vi "FGV_Undo Redo.vi"(7 "Action":T1, 8 "error in":errorcluster, 10 "State In":string, 11 "menu reference":refnum<k9>) -> (0 "error out":errorcluster, 1 "Have Changes":bool, 2 "State Out":string)   [LabVIEW 2020, in "lv_icon.lvlib" / "History.lvclass"]
doc: "Circular buffer used to maintain states of the icon for the purpose of being able to perform Undo and Redo.\n\nAfter initialization, it is expected the first \"Add\" will establish the initial condition."
uses:
  History.lvclass
  History.lvclass/History.ctl
  Undo Redo Action.ctl
panel:
  out "Had Roll Over":bool
  out "Available Redo":i32
  out "Available Undo":i32
  out "Current Pointer":i32
  out "Buffer":string[](array[string])
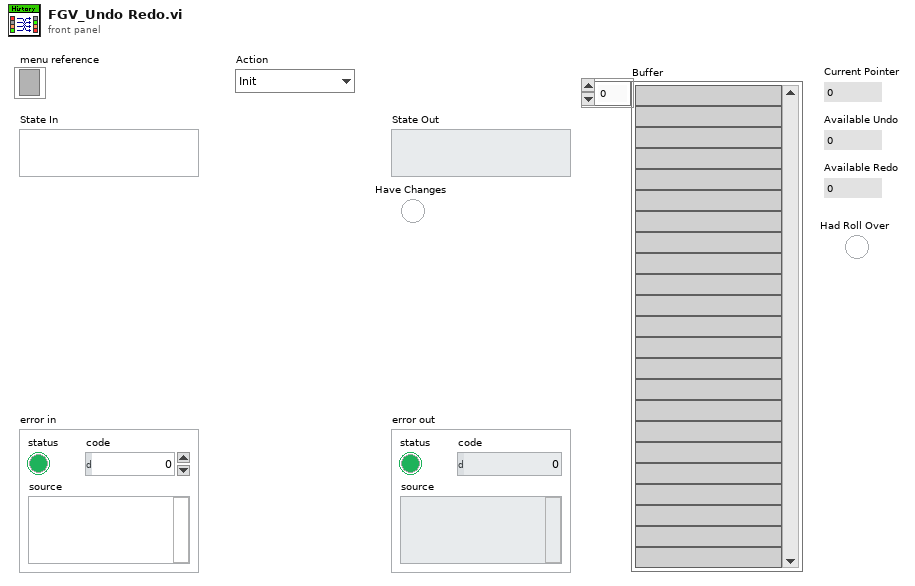
[diagram p1: front panel]
types:
  T1 = typedef "lv_icon.lvlib/History.lvclass/Undo Redo Action.ctl" = enum16{"Init", "Add", "Undo", "Redo", "Current State"}
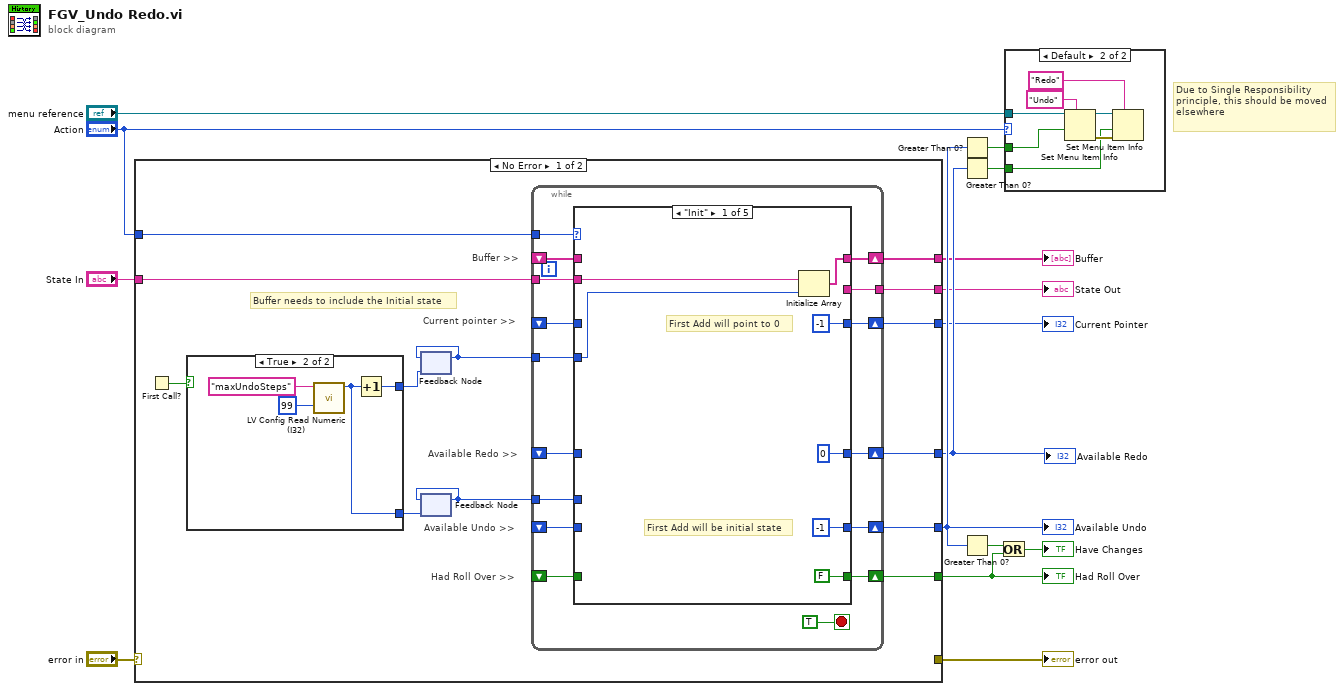
[diagram p0: block diagram]
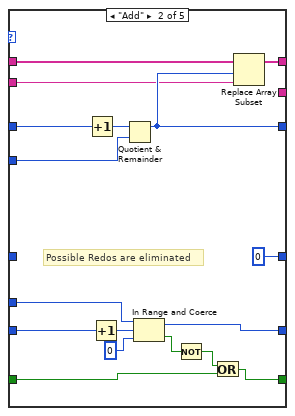
[diagram p3: hidden frame]
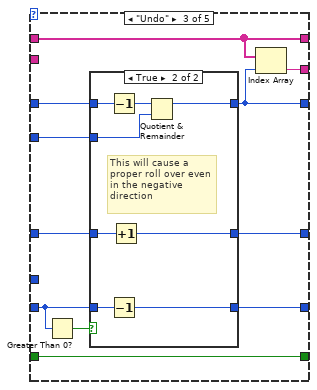
[diagram p4: hidden frame]
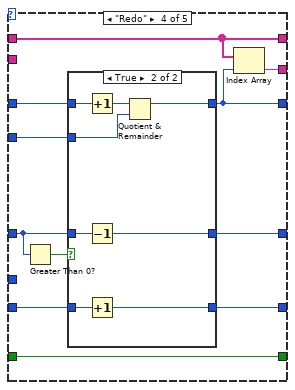
[diagram p6: hidden frame]
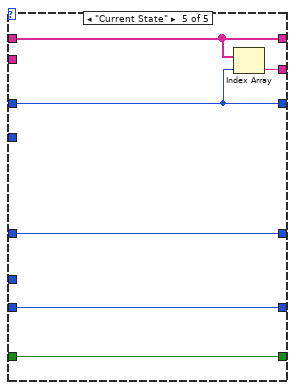
[diagram p8: hidden frame]
diagram:
  # "Due to Single Responsibility principle, this should be moved elsewhere"
  n1 = case shown="No Error" "error in" {
    selector: "error in" -> [_ w123]
    tunnel: [_ w123] -> w13
    tunnel: "Action" -> [w28 _]
    tunnel: "State In" -> [w27 _]
    tunnel: [w26 _] -> w3
    tunnel: [w23 _] -> w12
    tunnel: [w22 _] -> w1
    tunnel: [w20 _] -> w15
    tunnel: [w19 _] -> w2
    tunnel: [w16 _] -> w5
    frame No Error {
      # "Had Roll Over >>"
      # "Buffer needs to include the Initial state"
      # "Buffer >>"
      # "Available Undo >>"
      # "Available Redo >>"
      # "Current pointer >>"
      n2 = First Call?() -> (First Call?: T/F=w25:bool)
      n3 = case shown="True" w25 {
        tunnel: [_ w120] -> w21
        tunnel: [_ w119] -> w18
        frame False {
        }
        frame True {
          n4 = call <resource>:"LV Config Read Numeric (I32).vi"("default value"=99, "key"="maxUndoSteps") -> ("value"=w119:i32)  [unwired: 3 in, 2 out]
          n5 = Increment(x=w119) -> (x+1=w120:i32)
        }
      }
      n6 = feedback #1(w21) -> (w24:i32)
      n7 = feedback-in #1(w24) -> ()
      n8 = feedback #2(w18) -> (w17:i32)
      n9 = feedback-in #2(w17) -> ()
      n10 = while {
        tunnel: w28 -> [w43]
        shift-right: [w42] -> w19
        shift-left: _ -> [w41]
        tunnel: w27 -> [w40]
        shift-right: [w39] -> w22
        shift-left: _ -> [w38]
        shift-right: [w36] -> w23
        shift-left: _ -> [w37]
        tunnel: [w35] -> w26
        tunnel: w24 -> [w34]
        shift-right: [w32] -> w20
        shift-left: _ -> [w33]
        tunnel: w17 -> [w31]
        shift-right: [w29] -> w16
        shift-left: _ -> [w30]
        stop <- TRUE stop-if-true
        n11 = case shown="\"Init\"" w43 {
          tunnel: [w50 w68 w70 w100 w117] -> w42
          tunnel: w41 -> [_ w63 w70 w100 w117]
          tunnel: w40 -> [w48 w59 _ _ _]
          tunnel: [-1 w64 w77 w92 w116] -> w39
          tunnel: w38 -> [_ w67 w79 w98 w116]
          tunnel: w37 -> [_ _ w74 w96 w118]
          tunnel: [0 0 w73 w101 w118] -> w36
          tunnel: [_ _ w78 w99 w115] -> w35
          tunnel: w34 -> [w49 w58 w76 w95 _]
          tunnel: w33 -> [_ w56 w72 w94 w114]
          tunnel: [-1 w60 w71 w93 w114] -> w32
          tunnel: w31 -> [_ w57 _ _ _]
          tunnel: w30 -> [_ w55 w69 w91 w113]
          tunnel: [FALSE w54 w69 w91 w113] -> w29
          frame "Init" {
            # "First Add will be initial state"
            # "First Add will point to 0"
            n12 = Initialize Array(w48, w49) -> (w50:string[])
          }
          frame "Add" {
            # "Possible Redos are eliminated"
            n13 = Increment(x=w67) -> (x+1=w65:i32)
            n14 = Increment(x=w56) -> (x+1=w61:i32)
            n15 = Quotient & Remainder(x=w65, y=w58) -> (x-y*floor(x/y)=w64:i32)  [unwired: 1 out]
            n16 = In Range and Coerce(upper limit=w57, x=w61, lower limit=0) -> (coerced(x)=w60:i32, In Range?=w53:bool)
            n17 = Not(x=w53) -> (.not. x?=w52:bool)
            n18 = Or(x=w52, y=w55) -> (x .or. y?=w54:bool)
            n19 = Replace Array Subset(array=w63, new element=w59, index=w64) -> (w68:string[])
          }
          frame "Undo" {
            n20 = Greater Than 0?(x=w72) -> (x > 0?=w75:bool)
            n21 = case shown="True" w75 {
              tunnel: w79 -> [w82 w85]
              tunnel: [w82 w83] -> w77
              tunnel: w76 -> [_ w90]
              tunnel: w74 -> [w81 w89]
              tunnel: [w81 w88] -> w73
              tunnel: w72 -> [w80 w87]
              tunnel: [w80 w86] -> w71
              frame False {
              }
              frame True {
                # "This will cause a proper roll over even in the negative\ndirection"
                n22 = Decrement(x=w85) -> (x-1=w84:i32)
                n23 = Decrement(x=w87) -> (x-1=w86:i32)
                n24 = Increment(x=w89) -> (x+1=w88:i32)
                n25 = Quotient & Remainder(x=w84, y=w90) -> (x-y*floor(x/y)=w83:i32)  [unwired: 1 out]
              }
            }
            n26 = Index Array(array=w70, index=w77) -> (element=w78:string)
          }
          frame "Redo" {
            n27 = Greater Than 0?(x=w96) -> (x > 0?=w97:bool)
            n28 = case shown="True" w97 {
              tunnel: w96 -> [w104 w105]
              tunnel: [w104 w111] -> w101
              tunnel: w98 -> [w103 w110]
              tunnel: w95 -> [_ w112]
              tunnel: [w103 w108] -> w92
              tunnel: w94 -> [w102 w107]
              tunnel: [w102 w106] -> w93
              frame False {
              }
              frame True {
                n29 = Increment(x=w110) -> (x+1=w109:i32)
                n30 = Decrement(x=w105) -> (x-1=w111:i32)
                n31 = Increment(x=w107) -> (x+1=w106:i32)
                n32 = Quotient & Remainder(x=w109, y=w112) -> (x-y*floor(x/y)=w108:i32)  [unwired: 1 out]
              }
            }
            n33 = Index Array(array=w100, index=w92) -> (element=w99:string)
          }
          frame "Current State" {
            n34 = Index Array(array=w117, index=w116) -> (element=w115:string)
          }
        }
      }
    }
    frame Error {
    }
  }
  "error out" <- w13
  "State Out" <- w3
  "Buffer" <- w2
  "Current Pointer" <- w1
  "Available Undo" <- w15
  "Available Redo" <- w12
  "Had Roll Over" <- w5
  n35 = Greater Than 0?(x=w15) -> (x > 0?=w11:bool)
  n36 = Greater Than 0?(x=w12) -> (x > 0?=w8:bool)
  n37 = Greater Than 0?(x=w15) -> (x > 0?=w6:bool)
  n38 = Or(x=w6, y=w5) -> (x .or. y?=→"Have Changes":bool)
  n39 = case shown="Default" "Action" {
    tunnel: w11 -> [_ w126]
    tunnel: w8 -> [_ w125]
    tunnel: "menu reference" -> [_ w124]
    frame "Current State" {
    }
    frame Default {
      n40 = Set Menu Item Info(7:"Undo" ("Redo Menu Item"), 9:w126, 11:w124) -> (0:w130:errorcluster, 3:w129:refnum<k9>)  [unwired: 1 in, 3 out]
      n41 = Set Menu Item Info(7:"Redo" ("Undo Menu Item"), 8:w130, 9:w125, 11:w129) -> ()  [unwired: 5 out]
    }
  }
